vi "FitGaussian2 (SubVI).vi"(0 "x values":dbl[](array[numeric]), 1 "y values":dbl[](array[numeric]), 3 "method":T1 items=["Least Square", "Least Absolute Residual", "Bisquare"], 4 "confidence level":dbl=0.95, 5 "error in":errorcluster, 6 "Use all points":bool, 7 "Estimated mean":dbl, 8 "initial guess":T3={"initial amplitude"=nan, "initial center"=nan, "initial standard deviation"=nan, "offset"=nan}, 9 "Estimated width":dbl, 10 "parameter bounds":T2={"amp min"=-inf, "amp max"=inf, "center min"=-inf, "center max"=inf, "deviation min"=-inf, "deviation max"=inf, "offset min"=0.0, "offset max"=0.0}, 11 "Nsigma Low":dbl=4.0 format="%#_13g", 13 "Nsigma High":dbl=4.0 format="%#_13g") -> (14 "Plot with Gaussian fit":T4(graph), 15 "center":dbl, 16 "delta center":dbl, 17 "standard deviation":dbl, 18 "delta standard deviation":dbl, 19 "error out":errorcluster)   [LabVIEW 2016]
uses:
  <vilib>/Analysis/6fits.llb/Curve Fitting Criteria.ctl
  <vilib>/Analysis/6fits.llb/Confidence Interval (Gauss).vi
  <vilib>/Analysis/NI_AALPro.lvlib
panel:
  out "delta amplitude":dbl
  out "Best Gaussian Fit":dbl[](array[numeric])
  out "Selected x values":dbl[](array[numeric])
  out "Selected y values":dbl[](array[numeric])
  out "residue":dbl
  out "amplitude":dbl
  # "RESULTS"
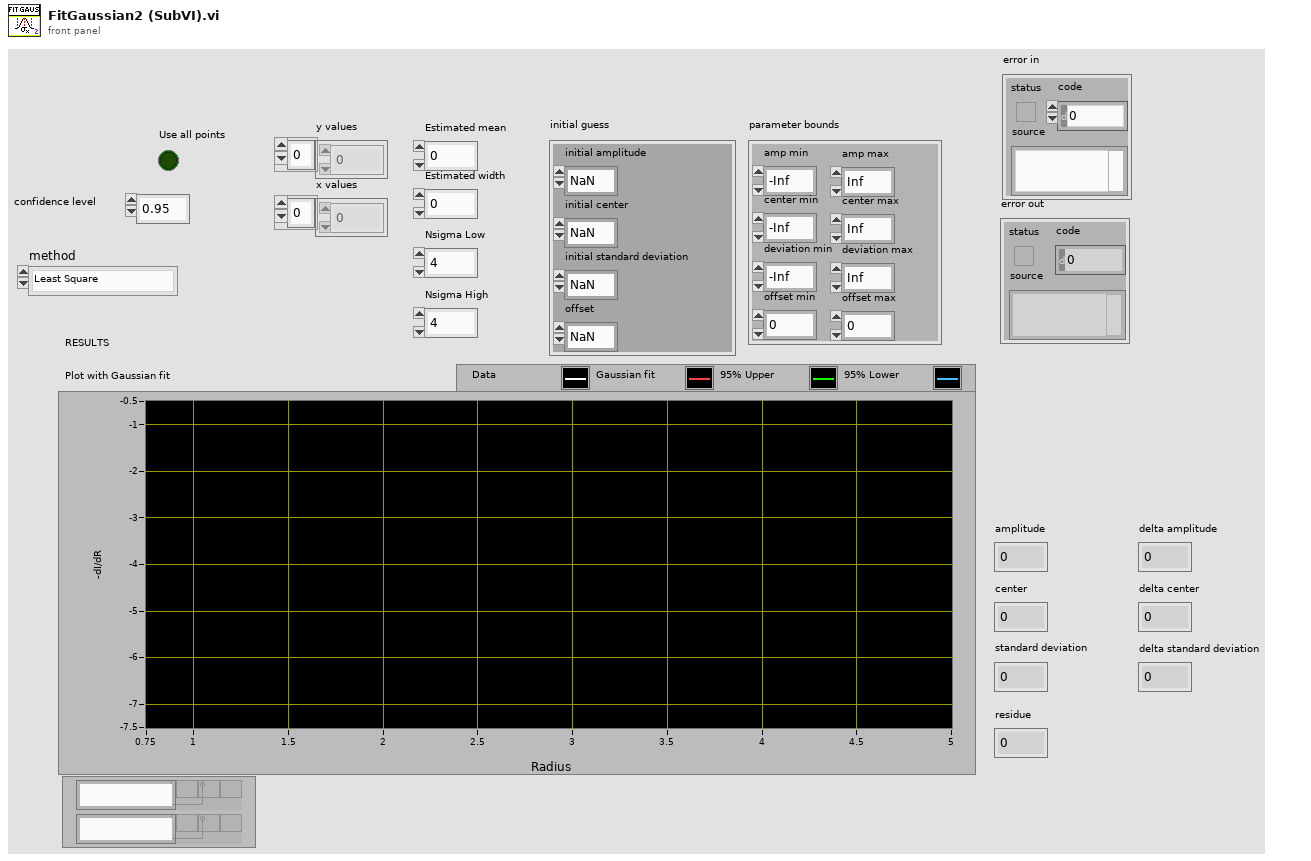
[diagram p1: front panel]
types:
  T1 = typedef "NI_AALPro.lvlib/Curve Fitting Criteria.ctl" = u16
  T2 = cluster{"amp min":dbl, "amp max":dbl, "center min":dbl, "center max":dbl, "deviation min":dbl, "deviation max":dbl, "offset min":dbl, "offset max":dbl}
  T3 = cluster{"initial amplitude":dbl, "initial center":dbl, "initial standard deviation":dbl, "offset":dbl}
  T4 = cluster{"Radius bins":dbl[], "Best Gaussian Fit":dbl[]}[]
  T5 = cluster{"Selected x values":dbl[], "Selected y values":dbl[]}
  T6 = cluster{"Selected x values":dbl[], "Best Gaussian Fit":dbl[]}
  T7 = cluster{"Selected x values":dbl[], "Upper Bound":dbl[]}
  T8 = cluster{"Selected x values":dbl[], "Lower Bound":dbl[]}
  T9 = cluster{"Selected x values":dbl[], "Lower Bound":dbl[]}[]
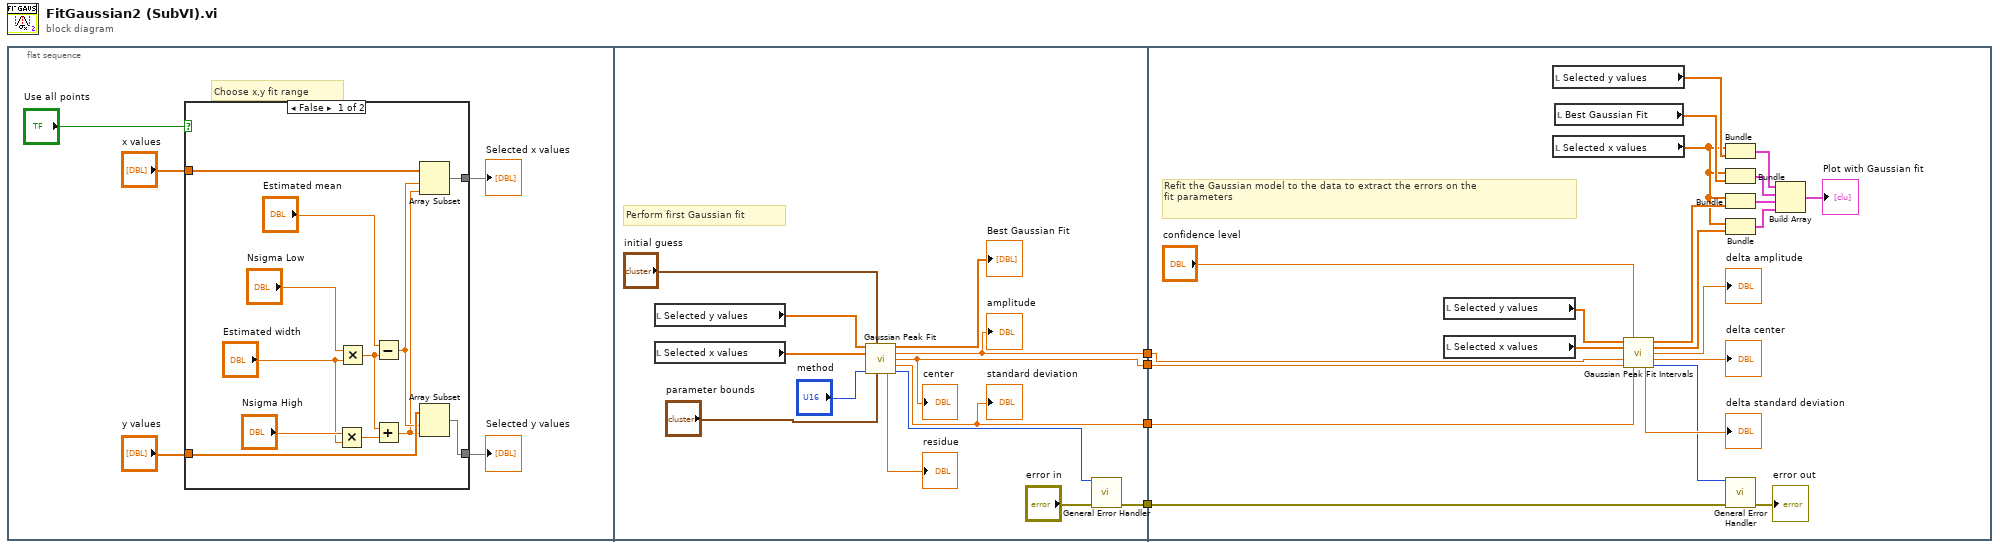
[diagram p0: block diagram]
diagram:
  n1 = flat-sequence {
    tunnel: [w31] -> w4
    tunnel: [w30] -> w3
    tunnel: [w28] -> w2
    tunnel: [w25] -> w1
    tunnel: w4 -> [w56]
    tunnel: w3 -> [w55]
    tunnel: w2 -> [w54]
    tunnel: w1 -> [w38]
    frame #0 {
      # "Choose x,y fit range"
      n2 = case shown="False" "Use all points" {
        tunnel: "y values" -> [w19 w22]
        tunnel: [w18 w22] -> w5
        tunnel: "x values" -> [w17 w23]
        tunnel: [w16 w23] -> w6
        frame False {
          n3 = Multiply(x="Nsigma High", y="Estimated width") -> (x*y=w11:dbl)
          n4 = Multiply(x="Nsigma Low", y="Estimated width") -> (x*y=w12:dbl)
          n5 = Subtract(x="Estimated mean", y=w12) -> (x-y=w15:dbl)
          n6 = Add(x=w12, y=w11) -> (x+y=w10:dbl)
          n7 = Array Subset(array=w17, index=w15, length=w10) -> (w16:dbl[])
          n8 = Array Subset(array=w19, index=w15, length=w10) -> (w18:dbl[])
        }
        frame True {
        }
      }
      "Selected y values" <- w5
      "Selected x values" <- w6
    }
    frame #1 {
      # "Perform first Gaussian fit"
      n9 = local read "Selected y values"() -> (w35:dbl[])
      n10 = local read "Selected x values"() -> (w34:dbl[])
      n11 = call <vilib>:"Gaussian Peak Fit.vi"("Y"=w35, "initial guess"="initial guess", "X"=w34, "method"="method", "parameter bounds"="parameter bounds") -> ("Best Gaussian Fit"=→"Best Gaussian Fit":dbl[], "amplitude"=w31:dbl, "center"=w30:dbl, "standard deviation"=w28:dbl, "residue"=→"residue":dbl, "error"=w26:i32)  [unwired: 4 in, 1 out]
      "center" <- w30
      "amplitude" <- w31
      "standard deviation" <- w28
      n12 = call <vilib>:"General Error Handler.vi"("[error code] (0)"=w26, "error in (no error)"="error in") -> ("error out"=w25:errorcluster)  [unwired: 9 in, 4 out]
    }
    frame #2 {
      # "Refit the Gaussian model to the data to extract the errors on the\nfit parameters"
      n13 = local read "Selected y values"() -> (w58:dbl[])
      n14 = local read "Selected x values"() -> (w57:dbl[])
      n15 = local read "Selected y values"() -> (w52:dbl[])
      n16 = local read "Selected x values"() -> (w44:dbl[])
      n17 = local read "Best Gaussian Fit"() -> (w51:dbl[])
      n18 = call-poly <vilib>:"Gaussian Peak Fit Intervals.vi"("Y"=w58, "confidence level"="confidence level", "X"=w57, "amplitude"=w56, "center"=w55, "standard deviation"=w54) -> ("Upper Bound"=w46:dbl[], "Lower Bound"=w45:dbl[], "delta amplitude"=→"delta amplitude":dbl, "delta center"=→"delta center":dbl, "delta standard deviation"=→"delta standard deviation":dbl, "error"=w39:i32)  [unwired: 4 in]
      n19 = Bundle("Selected x values"=w44, "Selected y values"=w52) -> (w50:T5)  [unwired: 1 in]
      n20 = Bundle("Selected x values"=w44, "Best Gaussian Fit"=w51) -> (w43:T6)  [unwired: 1 in]
      n21 = Bundle("Selected x values"=w44, "Upper Bound"=w46) -> (w42:T7)  [unwired: 1 in]
      n22 = Bundle("Selected x values"=w44, "Lower Bound"=w45) -> (w41:T8)  [unwired: 1 in]
      n23 = call <vilib>:"General Error Handler.vi"("[error code] (0)"=w39, "error in (no error)"=w38) -> ("error out"=→"error out":errorcluster)  [unwired: 9 in, 4 out]
      n24 = Build Array(w50, w43, w42, w41) -> (→"Plot with Gaussian fit":T9)
    }
  }
